vi "WBRT Motor Spinup.vi"(4 "Previous loop Right Command":dbl, 6 "Previous loop Left Command":dbl, 7 "Spin up time (s)":dbl=2.0, 8 "Time elapsed since Start":dbl, 9 "Current loop Right Command":dbl, 11 "Current loop Left Command":dbl) -> (0 "Right Command":dbl, 3 "Left Command":dbl)   [LabVIEW 2010]
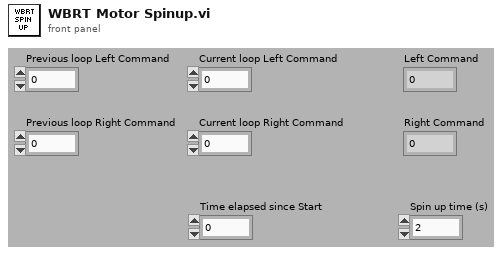
[diagram p1: front panel]
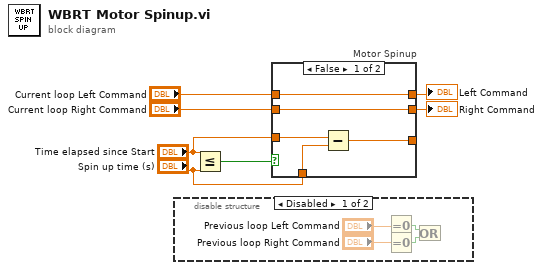
[diagram p0: block diagram]
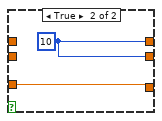
[diagram p3: hidden frame]
diagram:
  n1 = disable-structure shown="Disabled" {
    frame Disabled {
      n2 = Equal To 0?(x="Previous loop Left Command") -> (x = 0?=w11:bool)
      n3 = Equal To 0?(x="Previous loop Right Command") -> (x = 0?=w10:bool)
      n4 = Or(x=w11, y=w10) -> ()  [unwired: 1 out]
    }
    frame Enabled {
    }
  }
  n5 = Less Or Equal?(x="Time elapsed since Start", y="Spin up time (s)") -> (x <= y?=w3:bool)
  n6 = case "Motor Spinup" shown="False" w3 {
    tunnel: "Current loop Left Command" -> [w16 _]
    tunnel: "Current loop Right Command" -> [w15 _]
    tunnel: [w16 w18] -> w4
    tunnel: [w15 w18] -> w5
    tunnel: "Time elapsed since Start" -> [w14 w17]
    tunnel: "Spin up time (s)" -> [w13 _]
    tunnel: [w12 w17] -> _
    frame False {
      n7 = Subtract(x=w14, y=w13) -> (x-y=w12:dbl)
    }
    frame True {
      w18 = 10
    }
  }
  "Right Command" <- w5
  "Left Command" <- w4
